vi "Actor Teardown.vi"(10 "Error":errorcluster, 11 "Actor in":refnum<class "Actor.lvclass">) -> (0 "error out":errorcluster, 2 "Teardown?":bool, 3 "Actor out":refnum<class "Actor.lvclass">)   [LabVIEW 2021, in "LVCAM.lvlib" / "Actor.lvclass"]
uses:
  Actor.lvclass
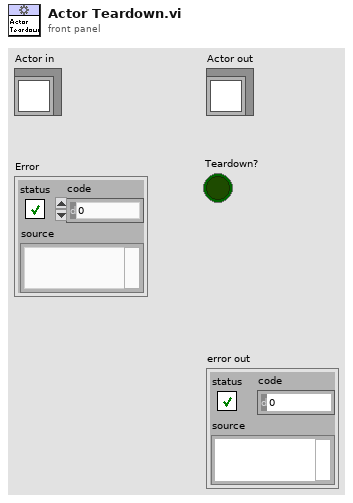
[diagram p1: front panel]
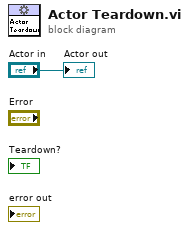
[diagram p0: block diagram]
diagram:
  "Actor out" <- "Actor in"
